vi "Show UI.vi"(0 "reference in":refnum<class "UI Manager.lvclass">, 2 "UI Type":T1, 5 "Error In":errorcluster) -> (14 "reference out":refnum<class "UI Manager.lvclass">, 19 "Error Out":errorcluster)   [LabVIEW 2024, in "UI Manager.lvclass"]
doc: "Pops up an new UI according to desired UI Type"
uses:
  UI Manager.lvclass
  UIType.ctl
  UI Manager.lvclass/UI Manager.ctl
panel:
  # "Connector Pane"
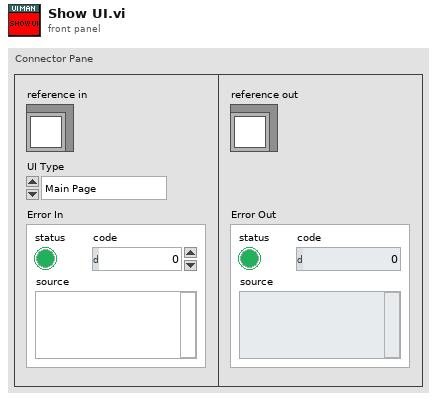
[diagram p1: front panel]
types:
  T1 = typedef "UIType.ctl" = enum16{"Main Page", "Settings Page", "Debugging Page"}
  T2 = typedef "UI Manager.lvclass/ObjectAttributes.ctl" = cluster{"Current Page":refnum<vi>}
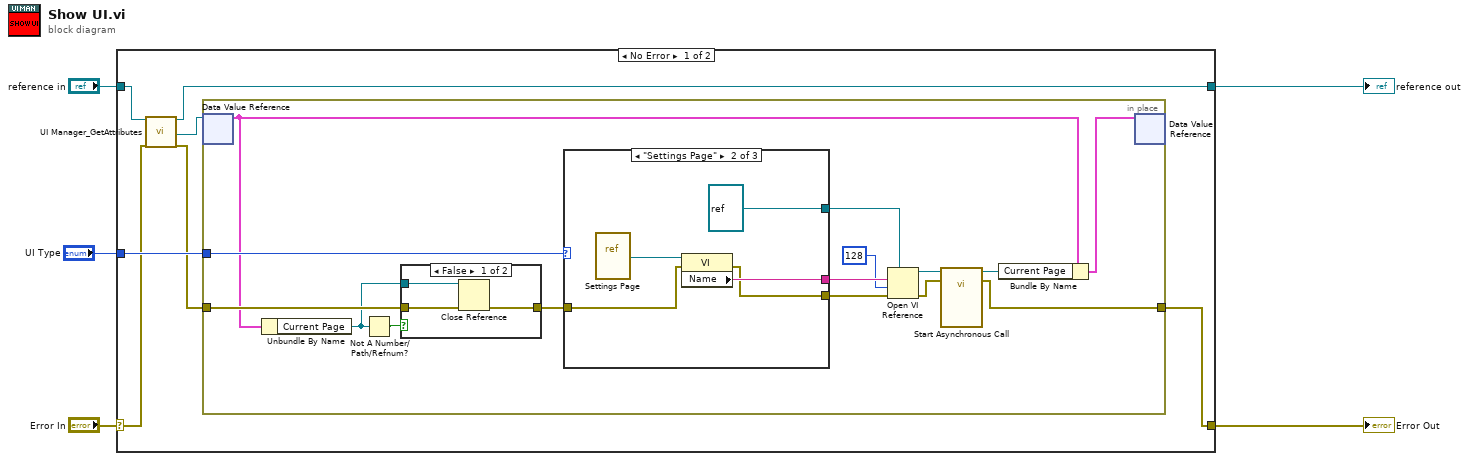
[diagram p0: block diagram]
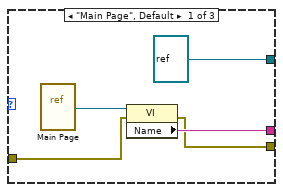
[diagram p3: hidden frame]
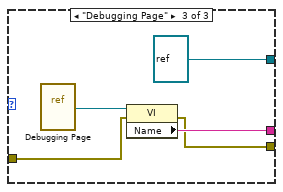
[diagram p4: hidden frame]
diagram:
  n1 = case shown="No Error" "Error In" {
    selector: "Error In" -> [w8 w48]
    tunnel: [w6 w48] -> w4
    tunnel: [w10 w47] -> w2
    tunnel: "reference in" -> [w11 w47]
    tunnel: "UI Type" -> [w12 _]
    frame No Error {
      n2 = call "UI Manager_GetAttributes.vi"("reference in"=w11, "Error In"=w8) -> ("reference out"=w10:refnum<class "UI Manager.lvclass">, "DataRef"=w7:refnum<data-value>, "Error Out"=w9:errorcluster)  [unwired: 14 in, 1 out]
      n3 = in-place {
        in-place-border: w12 -> [w27]
        in-place-border: w9 -> [w26]
        in-place-border: [w23] -> w6
        n4 = in-place-dvr #1(w7) -> (w25:T2)  [unwired: 1 out]
        n5 = Unbundle By Name(w25) -> ("Current Page"=w14:refnum<vi>)
        n6 = Not A Number/Path/Refnum?(number/path/refnum=w14) -> (NaN/Path/Refnum?=w13:bool)
        n7 = case shown="False" w13 {
          tunnel: w26 -> [w30 w31]
          tunnel: [w29 w31] -> w15
          tunnel: w14 -> [w28 _]
          frame False {
            n8 = Close Reference(reference=w28, error in (no error)=w30) -> (error out=w29:errorcluster)
          }
          frame True {
          }
        }
        n9 = case shown="\"Settings Page\"" w27 {
          tunnel: [refnum<vi> refnum ("type specifier VI Refnum (for type only)") refnum<vi> refnum ("type specifier VI Refnum (for type only)") refnum<vi> refnum ("type specifier VI Refnum (for type only)")] -> w22
          tunnel: [w34 w39 w44] -> w21
          tunnel: [w33 w38 w42] -> w17
          tunnel: w15 -> [w32 w37 w43]
          frame "Main Page", Default {
            n10 = vi-ref "Main Page.vi"() -> (w35:refnum<vi>)
            n11 = property class="VI"(reference=w35, error in=w32) -> (error out=w33:errorcluster, "Name"=w34:string)  [unwired: 1 out]
          }
          frame "Settings Page" {
            n12 = vi-ref "Settings Page.vi"() -> (w40:refnum<vi>)
            n13 = property class="VI"(reference=w40, error in=w37) -> (error out=w38:errorcluster, "Name"=w39:string)  [unwired: 1 out]
          }
          frame "Debugging Page" {
            n14 = vi-ref "Debugging Page.vi"() -> (w45:refnum<vi>)
            n15 = property class="VI"(reference=w45, error in=w43) -> (error out=w42:errorcluster, "Name"=w44:string)  [unwired: 1 out]
          }
        }
        n16 = Open VI Reference(type specifier VI Refnum (for type only)=w22, vi path=w21, options=128, error in (no error)=w17) -> (vi reference=w20:refnum<vi>, error out=w19:errorcluster)  [unwired: 2 in]
        n17 = call-by-ref "Start Asynchronous Call"(reference=w20, error in=w19) -> (reference out=w16:refnum<vi>, error out=w23:errorcluster)  [unwired: 1 in]
        n18 = Bundle By Name(cluster=w25, "Current Page"=w16) -> (w24:T2)
        n19 = in-place-dvr #1(w24) -> ()  [unwired: 2 out]
      }
    }
    frame Error {
    }
  }
  "Error Out" <- w4
  "reference out" <- w2
